vi "write galvo tasks.vi"(8 "error in (no error)":errorcluster, 11 "Waveform in":refnum<class "Waveform.lvclass">) -> (0 "error out":errorcluster, 3 "Waveform out":refnum<class "Waveform.lvclass">)   [LabVIEW 2012, in "Waveform.lvclass"]
uses:
  Waveform.lvclass
  Waveform.lvclass/Waveform.ctl
  <vilib>/DAQmx/write.llb/DAQmx Write (Analog 1D Wfm NChan NSamp).vi
  <vilib>/DAQmx/miscellaneous.llb/DAQmx Fill In Error Info.vi
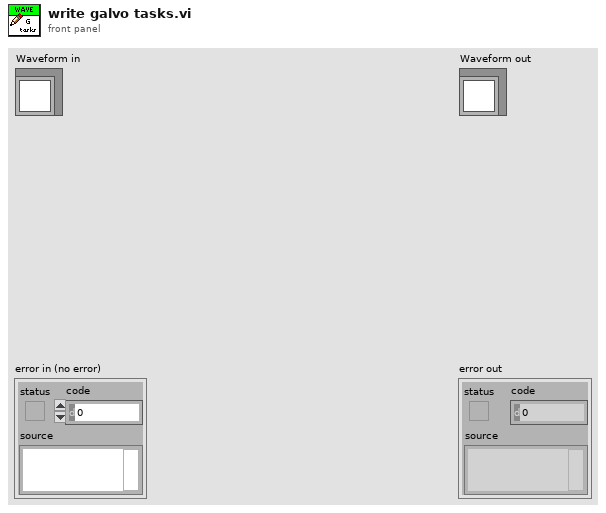
[diagram p1: front panel]
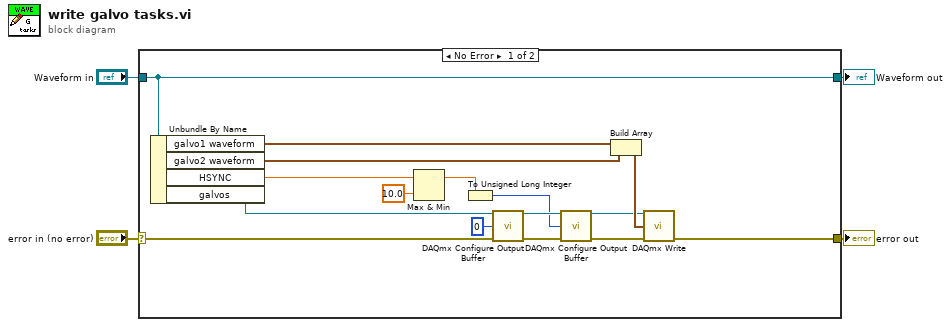
[diagram p0: block diagram]
diagram:
  n1 = case shown="No Error" "error in (no error)" {
    selector: "error in (no error)" -> [w9 w22]
    tunnel: [w17 w22] -> w3
    tunnel: [w20 w21] -> w1
    tunnel: "Waveform in" -> [w20 w21]
    frame No Error {
      n2 = Unbundle By Name(w20) -> ("galvo1 waveform"=w12:waveform(dbl), "galvo2 waveform"=w19:waveform(dbl), "HSYNC"=w6:dbl, "galvos"=w8:refnum<k21>)
      n3 = Max & Min(x=w6, y=10.0) -> (max(x,y)=w5:dbl)  [unwired: 1 out]
      n4 = To Unsigned Long Integer(number=w5) -> (unsigned 32bit integer=w10:u32)
      n5 = call <vilib>:"DAQmx Configure Output Buffer.vi"("task/channels in"=w8, "buffer size (in samples per channel)"=u32 0, "error in"=w9) -> ("task out"=w11:refnum<k21>, "error out"=w15:errorcluster)  [unwired: 11 in]
      n6 = call <vilib>:"DAQmx Configure Output Buffer.vi"("task/channels in"=w11, "buffer size (in samples per channel)"=w10, "error in"=w15) -> ("task out"=w13:refnum<k21>, "error out"=w14:errorcluster)  [unwired: 11 in]
      n7 = Build Array(w12, w19) -> (w18:waveform(dbl)[])
      n8 = call-poly <vilib>:"DAQmx Write.vi"("task/channels in"=w13, "data"=w18, "error in"=w14) -> ("error out"=w17:errorcluster)  [unwired: 10 in, 2 out]
    }
    frame Error {
    }
  }
  "error out" <- w3
  "Waveform out" <- w1
